vi "Create All Message Queues.vi"(8 "error in (no error)":errorcluster) -> (0 "error out":errorcluster, 3 "Message Queues out":T1)   [LabVIEW 2017, in "Message Queue.lvlib"]
doc: "This VI creates and initializes all the message queues for your application. If your application requires more than one message queue, right-click the \"Message Queues\" constant above and select Open Type Def. Add the new Message Queue(s) to the type definition, then initialize them in this VI."
uses:
  Message Queue.lvlib
  All Message Queues.ctl
  Message Cluster.ctl
  Enqueue Message (Single).vi
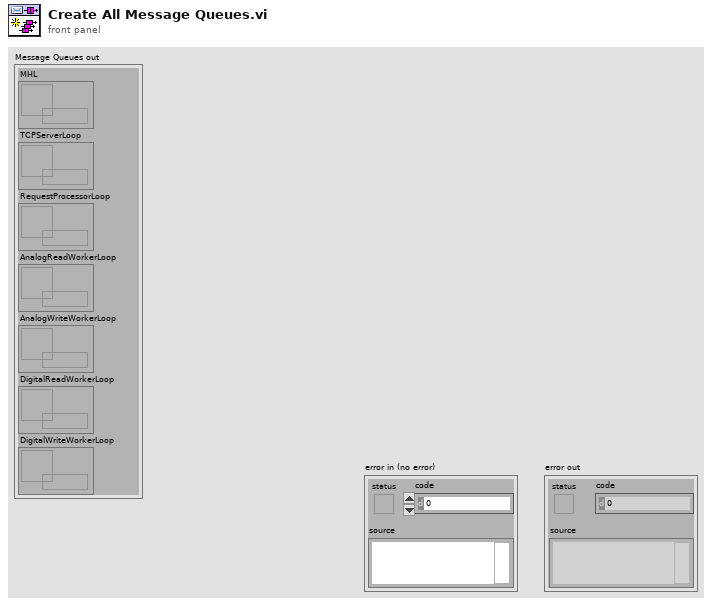
[diagram p1: front panel]
types:
  T1 = typedef "Message Queue.lvlib/All Message Queues.ctl" = cluster{"MHL":refnum<queue>, "TCPServerLoop":refnum<queue>, "RequestProcessorLoop":refnum<queue>, "AnalogReadWorkerLoop":refnum<queue>, "AnalogWriteWorkerLoop":refnum<queue>, "DigitalReadWorkerLoop":refnum<queue>, "DigitalWriteWorkerLoop":refnum<queue>}
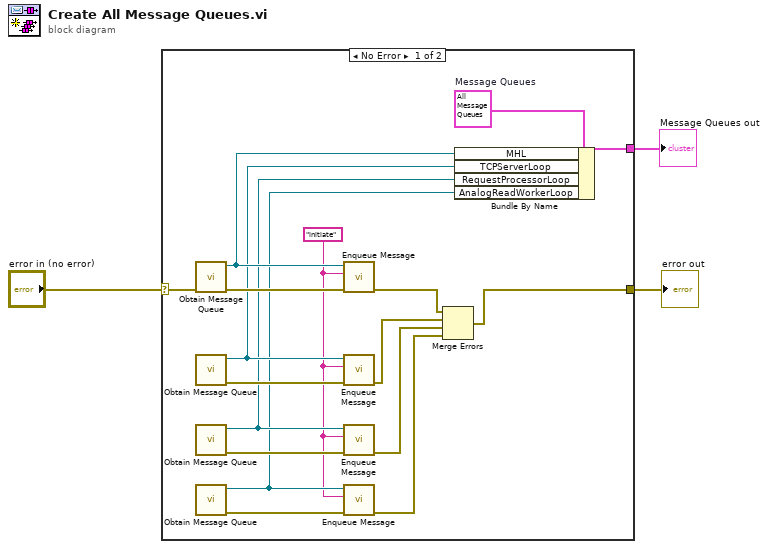
[diagram p0: block diagram]
diagram:
  n1 = case shown="No Error" "error in (no error)" {
    selector: "error in (no error)" -> [w18 w21]
    tunnel: [w4 w21] -> w3
    tunnel: [w19 _] -> w2
    frame No Error {
      w9 = "initiate" ("Message")
      w20 = T1 {"MHL"=refnum, "TCPServerLoop"=refnum, "RequestProcessorLoop"=refnum, "AnalogReadWorkerLoop"=refnum, "AnalogWriteWorkerLoop"=refnum, "DigitalReadWorkerLoop"=refnum, "DigitalWriteWorkerLoop"=refnum}  # Message Queues
      n2 = call "Obtain Message Queue.vi"("error in (no error)"=w18) -> ("error out"=w17:errorcluster, "Message Queue"=w16:refnum<queue>)  [unwired: 9 in]
      n3 = call "Obtain Message Queue.vi"() -> ("error out"=w15:errorcluster, "Message Queue"=w14:refnum<queue>)  [unwired: 10 in]
      n4 = call "Obtain Message Queue.vi"() -> ("error out"=w13:errorcluster, "Message Queue"=w12:refnum<queue>)  [unwired: 10 in]
      n5 = call "Obtain Message Queue.vi"() -> ("error out"=w11:errorcluster, "Message Queue"=w10:refnum<queue>)  [unwired: 10 in]
      n6 = call-poly "Enqueue Message.vi"("error in (no error)"=w17, "Message"=w9, "Message Queue"=w16) -> ("error out"=w8:errorcluster)  [unwired: 7 in, 1 out]
      n7 = call-poly "Enqueue Message.vi"("error in (no error)"=w15, "Message"=w9, "Message Queue"=w14) -> ("error out"=w7:errorcluster)  [unwired: 7 in, 1 out]
      n8 = call-poly "Enqueue Message.vi"("error in (no error)"=w13, "Message"=w9, "Message Queue"=w12) -> ("error out"=w6:errorcluster)  [unwired: 7 in, 1 out]
      n9 = call-poly "Enqueue Message.vi"("error in (no error)"=w11, "Message"=w9, "Message Queue"=w10) -> ("error out"=w5:errorcluster)  [unwired: 7 in, 1 out]
      n10 = Merge Errors(w8, w7, w6, w5) -> (w4:errorcluster)
      n11 = Bundle By Name(cluster=w20, "MHL"=w16, "TCPServerLoop"=w14, "RequestProcessorLoop"=w12, "AnalogReadWorkerLoop"=w10) -> (w19:T1)
    }
    frame Error {
    }
  }
  "Message Queues out" <- w2
  "error out" <- w3
